vi "Thermocouple (with OTCD) - Continuous Input.vi"() -> ()   [LabVIEW 2022 SP3]
doc: "This example demonstrates how to continuously acquire temperature measurements using a DAQmx device. It also includes open Thermocouple detection for devices that support that feature.\n\nFor instructions on how to connect your signals to the DAQ device, refer to your device documentation."
uses:
  <vilib>/Utility/error.llb/DialogType.ctl
  <vilib>/DAQmx/read.llb/DAQmx Read (Analog 1D Wfm NChan NSamp).vi
  <vilib>/DAQmx/create/channels.llb/DAQmx Create Channel (AI-Temperature-Thermocouple).vi
  <vilib>/DAQmx/configure/timing.llb/DAQmx Timing (Sample Clock).vi
  <vilib>/DAQmx/miscellaneous.llb/DAQmx Fill In Error Info.vi
  <resource>/objmgr/daqmx.rc
panel:
  in  "Thermocouple Type":i32(ring)=10072 items=["J"=10072, "K"=10073, "N"=10077, "R"=10082, "S"=10085, "T"=10086, "B"=10047, "E"=10055]
  in  "Open TC Status Table":string[][](table)=[["", ""]] caption="Open Thermocouple \nStatus Table"
  out "Open Thermocouple \nChannels":string[](array[string])
  out "Open Thermocouples?":bool
  in  "Perform Lead Offset Nulling**":bool
  in  "Disable Open TC Detection?*":bool
  in  "CJC Channel":refnum<k21>
  in  "CJC Value":dbl=25.0 format="%0.2f"
  in  "CJC Source":i32(ring)=10116 items=["Built-In"=10200, "Constant Value"=10116, "Channel"=10113]
  in  "Stop":bool
  out "Waveform Graph":waveform(dbl)[](graph)
  in  "Samples per Loop":i32=100
  in  "Sample Rate":dbl=1000.0
  in  "Sample Clock Source":tag="OnboardClock"
  in  "Max Value (deg C)":dbl=100.0
  in  "Min Value (deg C)":dbl
  in  "Physical Channel":tag="Dev1/ai0"
  out "Actual Sample Rate":dbl format="%0.2f"
  # "Channel Settings"
  # "Acquired Data"
  # "Timing Settings"
  # "Open Thermocouple Detection Settings"
  # "* Some devices do not support disabling open thermocouple detection, such as the NI 9213.\n** Only certain devices support performing lead offset nulling, such as the NI 9214."
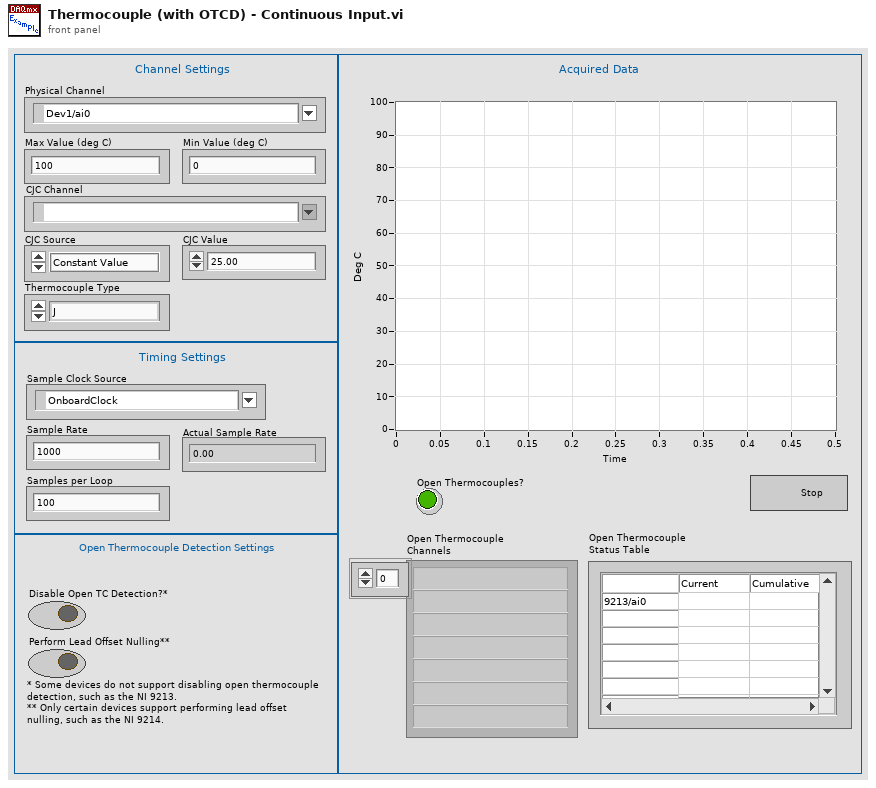
[diagram p1: front panel]
types:
  T1 = typedef "DialogType.ctl" = u16
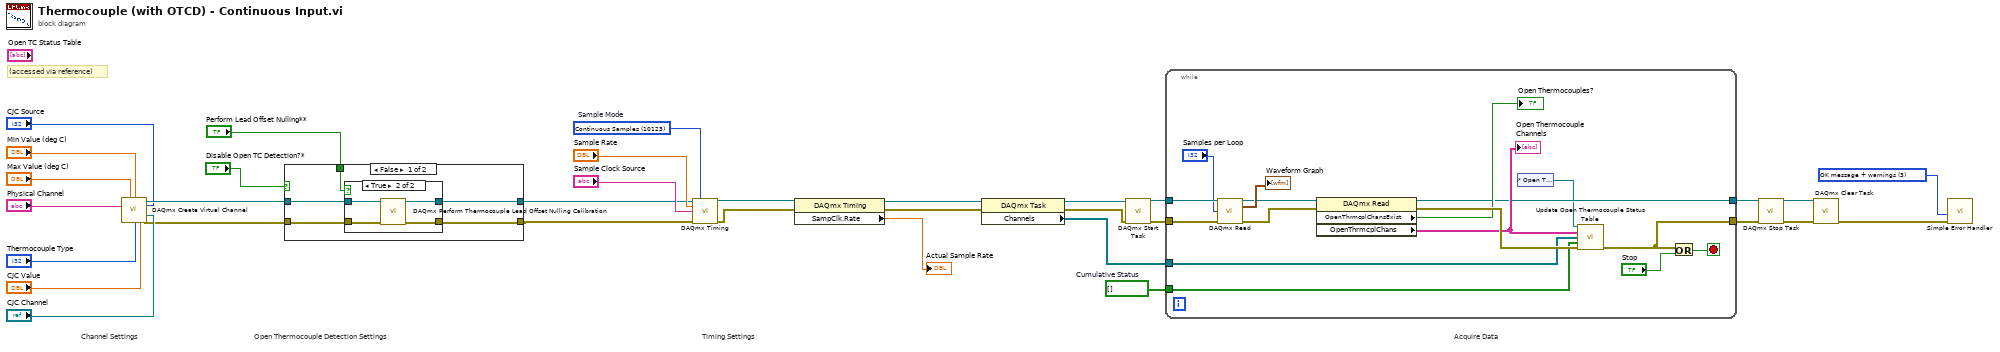
[diagram p0: block diagram]
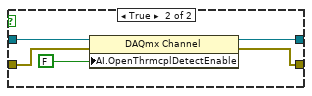
[diagram p3: hidden frame]
diagram:
  w5 = T1 3 items=["no dialog", "OK message", "continue or stop message", "OK message + warnings", "continue/stop + warnings"] ("type of dialog (OK msg:1)")
  w13 = bool[] []  # Cumulative Status
  w31 = 10123 items=["Finite Samples"=10178, "Continuous Samples"=10123, "Hardware Timed Single Point"=12522]  # Sample Mode
  # "Open Thermocouple Detection Settings"
  # "(accessed via reference)"
  # "Acquire Data"
  # "Timing Settings"
  # "Channel Settings"
  n1 = call-poly <vilib>:"DAQmx Create Virtual Channel.vi"("maximum value"="Max Value (deg C)", "minimum value"="Min Value (deg C)", "physical channels"="Physical Channel", "cjc source"="CJC Source", "cjc channel"="CJC Channel", "thermocouple type"="Thermocouple Type", "cjc value"="CJC Value") -> ("task out"=w16:refnum<k21>, "error out"=w17:errorcluster)  [unwired: 7 in]
  n2 = case shown="False" "Disable Open TC Detection?*" {
    tunnel: w16 -> [w38 w48]
    tunnel: w17 -> [w37 w47]
    tunnel: [w35 w46] -> w15
    tunnel: [w36 w45] -> w14
    tunnel: "Perform Lead Offset Nulling**" -> [w34 _]
    frame False {
      n3 = case shown="True" w34 {
        tunnel: w38 -> [w40 w44]
        tunnel: w37 -> [w39 w43]
        tunnel: [w39 w42] -> w36
        tunnel: [w40 w41] -> w35
        frame False {
        }
        frame True {
          n4 = call <vilib>:"DAQmx Perform Thermocouple Lead Offset Nulling Calibration.vi"("task/channels in"=w44, "error in"=w43) -> ("task out"=w41:refnum<k21>, "error out"=w42:errorcluster)  [unwired: 12 in]
        }
      }
    }
    frame True {
      n5 = property class="DAQmx Channel"(reference=w48, error in=w47, "AI.OpenThrmcplDetectEnable"=FALSE) -> (reference out=w46:refnum<k21>, error out=w45:errorcluster)
    }
  }
  n6 = call-poly <vilib>:"DAQmx Timing.vi"("task/channels in"=w15, "sample mode"=w31, "rate"="Sample Rate", "source"="Sample Clock Source", "error in"=w14) -> ("task out"=w33:refnum<k21>, "error out"=w32:errorcluster)  [unwired: 9 in]
  n7 = property class="DAQmx Timing"(reference=w33, error in=w32) -> (reference out=w12:refnum<k21>, error out=w11:errorcluster, "SampClk.Rate"=→"Actual Sample Rate":dbl)
  n8 = property class="DAQmx Task"(reference=w12, error in=w11) -> (reference out=w10:refnum<k21>, error out=w9:errorcluster, "Channels"=w8:refnum<k21>[])
  n9 = call <vilib>:"DAQmx Start Task.vi"("task/channels in"=w10, "error in"=w9) -> ("task out"=w30:refnum<k21>, "error out"=w29:errorcluster)  [unwired: 12 in]
  n10 = while {
    tunnel: w30 -> [w64]
    tunnel: w29 -> [w63]
    tunnel: [w54] -> w3
    tunnel: [w51] -> w4
    tunnel: w13 -> [w53]
    tunnel: w8 -> [w52]
    stop <- w62 stop-if-true
    n11 = call-poly <vilib>:"DAQmx Read.vi"("task/channels in"=w64, "number of samples per channel"="Samples per Loop", "error in"=w63) -> ("task out"=w58:refnum<k21>, "data"=→"Waveform Graph":waveform(dbl)[], "error out"=w57:errorcluster)  [unwired: 10 in]
    n12 = property class="DAQmx Read"(reference=w58, error in=w57) -> (reference out=w51:refnum<k21>, error out=w65:errorcluster, "OpenThrmcplChansExist"=→"Open Thermocouples?":bool, "OpenThrmcplChans"=w55:string[])
    "Open Thermocouple \nChannels" <- w55
    n13 = control-ref of="Open TC Status Table"() -> (w50:refnum<vi>)
    n14 = call "Update Open Thermocouple Status Table.vi"("Open Thermocouple Status Table"=w50, "Open Thermocouple Channels"=w55, "Task Channels"=w52, "Cumulative Status In"=w53, "Error In"=w65) -> ("Error Out"=w54:errorcluster)  [unwired: 9 in, 1 out]
    n15 = Or(x=w54, y="Stop") -> (x .or. y?=w62:bool)
  }
  n16 = call <vilib>:"DAQmx Stop Task.vi"("task/channels in"=w4, "error in"=w3) -> ("task out"=w2:refnum<k21>, "error out"=w1:errorcluster)  [unwired: 12 in]
  n17 = call <vilib>:"DAQmx Clear Task.vi"("task in"=w2, "error in"=w1) -> ("error out"=w28:errorcluster)  [unwired: 13 in]
  n18 = call <vilib>:"Simple Error Handler.vi"("type of dialog (OK msg:1)"=w5, "error in (no error)"=w28) -> ()  [unwired: 3 in, 5 out]
